vi "Creators Self Queue.vi"(9 "Priority?":bool, 10 "Msg Strategy":refnum<class "Msg Strategy.lvclass">, 11 "Base Event in":refnum<class "Base Event.lvclass">) -> (3 "Base Event out":refnum<class "Base Event.lvclass">)   [LabVIEW 2021, in "jettl.lvlib" / "Base Event.lvlib" / "Base Event.lvclass"]
uses:
  Base Event.lvclass
  Queue Mailbox/Queue Mailbox.lvlib
  Self Queue/Self Queue.lvlib
  Msg Strategy/Msg Strategy.lvclass
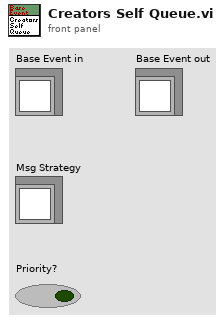
[diagram p1: front panel]
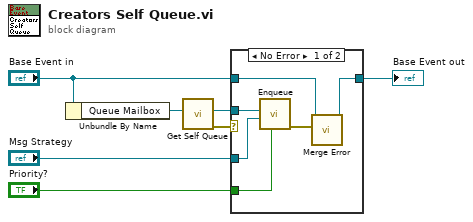
[diagram p0: block diagram]
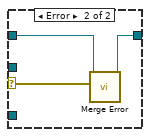
[diagram p2: hidden frame]
diagram:
  n1 = Unbundle By Name("Base Event in") -> ("Queue Mailbox"=w5:refnum<data-value>)
  n2 = call "Get Self Queue.vi"("Queue Mailbox"=w5) -> ("error out"=w6:errorcluster, "Self Queue"=w7:refnum<data-value>)  [unwired: 9 in]
  n3 = case shown="No Error" w6 {
    selector: w6 -> [_ w15]
    tunnel: "Priority?" -> [w12 _]
    tunnel: "Msg Strategy" -> [w11 _]
    tunnel: "Base Event in" -> [w10 w14]
    tunnel: [w9 w16] -> w1
    tunnel: w7 -> [w8 _]
    frame No Error {
      n4 = call "Enqueue.vi"("Priority?"=w12, "Msg Strategy"=w11, "Self Queue"=w8) -> ("error out"=w13:errorcluster)  [unwired: 8 in]
      n5 = call-dynamic "Merge Error.vi"("Error"=w13, "Base Event in"=w10) -> ("Base Event out"=w9:refnum<class "Base Event.lvclass">)  [unwired: 9 in]
    }
    frame Error {
      n6 = call-dynamic "Merge Error.vi"("Error"=w15, "Base Event in"=w14) -> ("Base Event out"=w16:refnum<class "Base Event.lvclass">)  [unwired: 9 in]
    }
  }
  "Base Event out" <- w1
